vi "Car Position Desired Update.vi"(8 "error in (no error)":errorcluster, 10 "Car Position Desired":u8, 11 "iCar Position Monitor Model in":refnum<class "iCar Position Monitor Model.lvclass">) -> (0 "error out":errorcluster, 3 "iCar Position Monitor Model out":refnum<class "iCar Position Monitor Model.lvclass">)   [LabVIEW 2019, in "iCar Position Monitor Model.lvclass"]
uses:
  <vilib>/gpm_packages/@cs/Car-wash/Source/iCar Position Monitor Model/iCar Position Monitor Model/iCar Position Monitor Model.lvclass
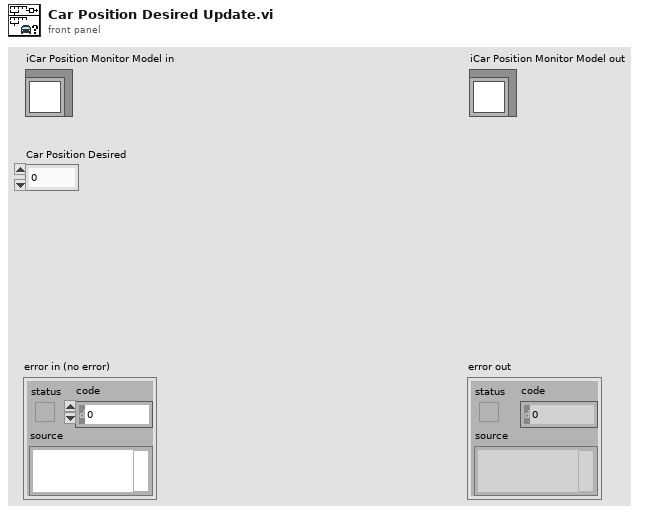
[diagram p1: front panel]
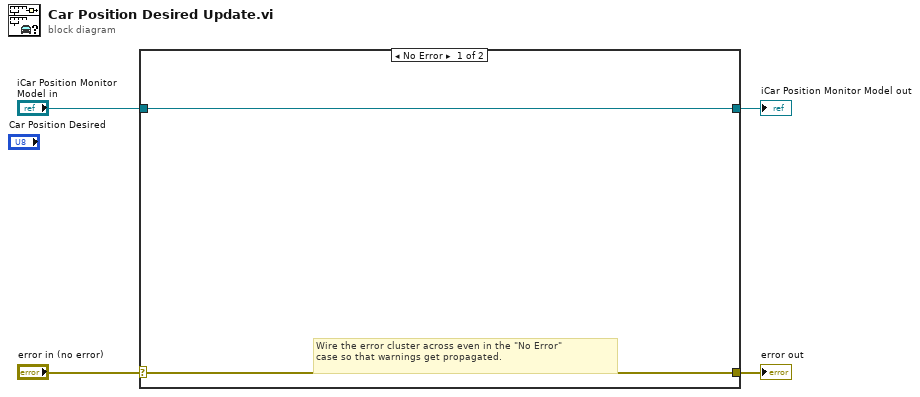
[diagram p0: block diagram]
diagram:
  n1 = case shown="No Error" "error in (no error)" {
    selector: "error in (no error)" -> [w5 w8]
    tunnel: [w5 w8] -> w3
    tunnel: [w6 w7] -> w1
    tunnel: "iCar Position Monitor Model in" -> [w6 w7]
    frame No Error {
      # "Wire the error cluster across even in the \"No Error\"\ncase so that warnings get propagated."
    }
    frame Error {
    }
  }
  "error out" <- w3
  "iCar Position Monitor Model out" <- w1
